vi "Track Registers and Write RFFE Waveform.vi"(0 "Semiconductor Module Context":T3, 1 "Pins":string[](array[string])=["CLK", "SDA"], 3 "Reg_Map":string[][](array[string])=[["Reg Addr(0x00)", "7", "6", "5", "4", "3", "2", "1", "0"], ["0", "SPARE", "RF3_SH", "RF2_SH", "RF1_SH", "SPARE", "RF3_RFC", "RF2_RFC", "RF1_RFC"], ["1", "SPARE[7:0]", "", "", "", "", "", "", ""], ["2", "VVAR_EN", "LCM_EN", "RFC_SH", "SPARE", "VARACTOR[3:0]", "", "", ""], ["3", "SW_CTRL1_VIRTUAL[7:0]", "", "", "", "", "", "", ""], ["4", "SW_CTRL1_SWAP", "SW_CTRL1_RBSHIFT[2:0]", "", "", "SW_CTRL1_VSID[3:0]", "", "", ""], ["5", "REG_00_VIRTUAL_MASK[7:0]", "", "", "", "", "", "", ""], ["6", "LOCK_STATUS[1:0]", "", "CLK_DITHER", "FUSES_BURNED", "CLK_IDAC_CAL[3:0]", "", "", ""], ["7", "SPARE[2:0]", "", "", "ODFT_TRIM[4:0]", "", "", "", ""], ["8", "SPARE[2:0]", "", "", "HV_TRIM[4:0]", "", "", "", ""], ["9", "TEST_MUX[2:0]", "", "", "SPARE[1:0]", "", "MEMS_BG_TC[1:0]", "", "MEMSCP_RCM"], ["A", "CP_BOOST_OVRD_EN", "SPARE[2:0]", "", "", "PS_OFF_TIMER[1:0]", "", "PS_ON_TIMER[1:0]", ""], ["0", "", "", "", "", "", "", "", ""], ["D", "Reserved[1:0]", "", "WD_HI_EVENT_CNT[5:0]", "", "", "", "", ""], ["E", "VERSION_ID[7:0]", "", "", "", "", "", "", ""], ["F", "Reserved", "COUNT_200_LSB[6:0]", "", "", "", "", "", ""], ["10", "CLK_DIV2_EN", "Spare", "ODFT_EN", "HV_HYST[4:0]", "", "", "", ""], ["0", "", "", "", "", "", "", "", ""], ["12", "SHORT_FUSE", "FUSE_BURN", "STROBE_EN", "VIO_OK", "RTH[1:0]", "", "FUSE_LOAD_MAN_EN", "FUSE_LOAD"], ["13", "RR_ACK_EN", "Reserved", "ACK_POSITION[1:0]", "", "SuBUS_DRIVE_STRENGTH[3:0]", "", "", ""], ["14", "TM_IO_EN", "TM_IO_SEL", "SuBUS_OVS[1:0]", "", "Reserved[3:0]", "", "", ""], ["15", "Reserved[4:0]", "", "", "", "", "SuBUS_VERSION_PRESENT", "SuBUS_VOLTAGE", "SuBUS_FLAVOR_DEF"], ["16", "PROG_STROBE1_DUR[7:0]", "", "", "", "", "", "", ""], ["17", "PROG_STROBE0_DUR[7:0]", "", "", "", "", "", "", ""], ["18", "Reserved[2:0]", "", "", "EFUSE_SINGLE_ADDR_SEL[4:0]", "", "", "", ""], ["19", "POLL_ADR[4:0]", "", "", "", "", "POLL_BC[2:0]", "", ""], ["1A", "SOFTWARE_RESET", "Reserved[6:0]", "", "", "", "", "", ""], ["1B", "Reserved[7:0]", "", "", "", "", "", "", ""], ["1C", "PWR_MODE_1", "PWR_MODE_0", "TRIGGER_MASK[2:0]", "", "", "TRIGGER[2:0]", "", ""], ["1D", "PRODUCT_ID[7:0]", "", "", "", "", "", "", ""], ["1E", "MANUFACTURER_ID_LSB[7:0]", "", "", "", "", "", "", ""], ["1F", "MANUFACTURER_ID_MSB[3:0]", "", "", "", "USID[3:0]", "", "", ""]], 4 "Master_Register_Data_Array_In":T1 {"Address" format="%.0x"}, 5 "Error In":errorcluster, 6 "Reg_Map_Bit_Name":string="HV_TRIM", 8 "Script_Functions":enum16{"Reg_Write", "Bit_Write"}(ring), 10 "USID":T4 max=15, 11 "Reg_Address_Data":T2={"Address"=81, "Data"=0} {"Address" format="%.0x"}) -> (14 "Semiconductor Module Context Out":T3, 15 "Master_Register_Data_Array_Out":T1 {"Address" format="%.0x"}, 19 "Error Out":errorcluster)   [LabVIEW 2013]
uses:
  Controls/Master_Reg_Data_Array.ctl
  Controls/Reg_Address_Data.ctl
  Controls/USID.ctl
  <vilib>/NI_TestStand_SemiconductorModule/NI_TestStand_Semiconductor_Module.lvlibp/PinMap/General/SemiconductorModuleContext.ctl
  <vilib>/NI_TestStand_SemiconductorModule/NI_TestStand_Semiconductor_Module.lvlibp
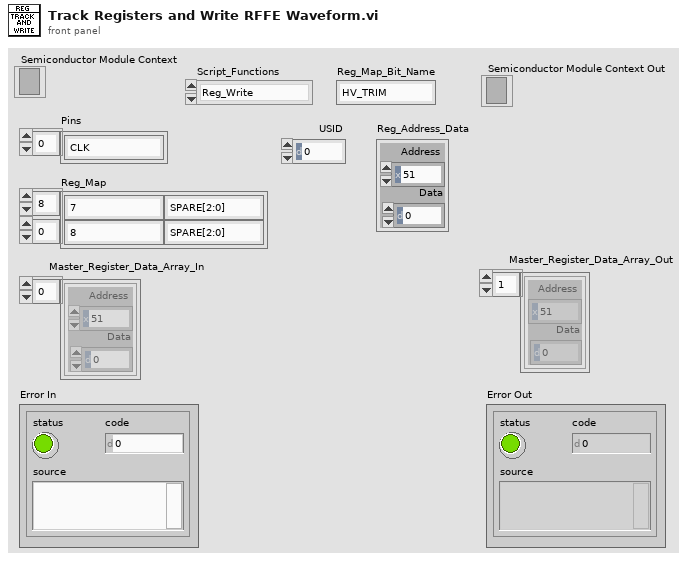
[diagram p1: front panel]
types:
  T1 = typedef "Master_Reg_Data_Array.ctl" = T2[]
  T2 = typedef "Reg_Address_Data.ctl" = cluster{"Address":u8, "Data":u8}
  T3 = typedef "NI_TestStand_Semiconductor_Module.lvlibp/SemiconductorModuleContext.ctl" = refnum<k7>
  T4 = typedef "USID.ctl" = u8
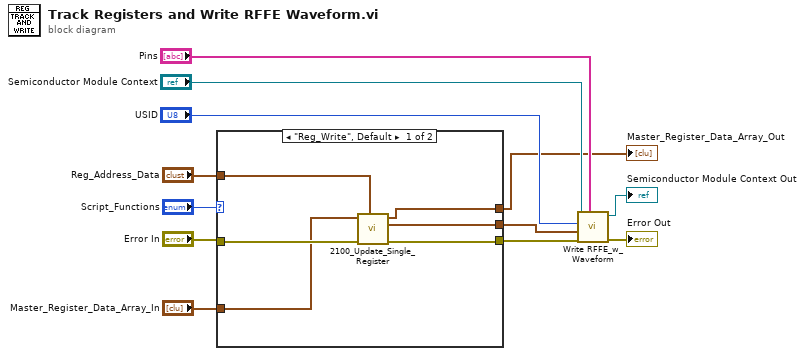
[diagram p0: block diagram]
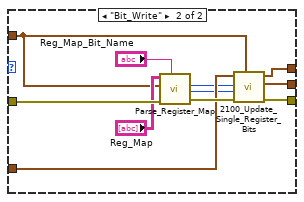
[diagram p2: hidden frame]
diagram:
  n1 = case shown="\"Reg_Write\", Default" "Script_Functions" {
    tunnel: "Error In" -> [w18 w29]
    tunnel: "Reg_Address_Data" -> [w15 w25]
    tunnel: "Master_Register_Data_Array_In" -> [w16 w24]
    tunnel: [w17 w21] -> w4
    tunnel: [w14 w20] -> w3
    tunnel: [w13 w19] -> w1
    frame "Reg_Write", Default {
      n2 = call "2100_Update_Single_Register.vi"("Reg_Address_Data"=w15, "Error In"=w18, "Master_Register_Data_Array_In"=w16) -> ("Error Out"=w17:errorcluster, "Single_Reg_Address_Data Out"=w14:T2, "Master_Register_Data_Array_Out"=w13:T1)  [unwired: 6 in]
    }
    frame "Bit_Write" {
      n3 = call "Parse_Register_Map.vi"("Reg_Map_Bit_Name"="Reg_Map_Bit_Name", "Error In"=w29, "Reg_Address_Data"=w25, "Reg_Map"="Reg_Map") -> ("Error Out"=w26:errorcluster, "Length"=w22:u8, "LSB"=w23:u8)  [unwired: 4 in, 1 out]
      n4 = call "2100_Update_Single_Register_Bits.vi"("Reg_Address_Data"=w25, "Error In"=w26, "Length"=w22, "LSB"=w23, "Master_Register_Data_Array_In"=w24) -> ("Error Out"=w21:errorcluster, "Single_Reg_Address_Data Out"=w20:T2, "Master_Register_Data_Array_Out"=w19:T1)  [unwired: 4 in]
    }
  }
  "Master_Register_Data_Array_Out" <- w1
  n5 = call "Write RFFE_w_Waveform.vi"("Pins"="Pins", "error in (no error)"=w4, "Reg_Address_Data"=w3, "USID"="USID", "Semiconductor Module Context"="Semiconductor Module Context") -> ("error out"=→"Error Out":errorcluster, "Semiconductor Module Context Out"=→"Semiconductor Module Context Out":T3)  [unwired: 5 in]
